vi "Reshape_DDcontroller.vi"(11 "path refs":path) -> (0 "error out":errorcluster, 3 "output array":dbl[](array[numeric]))   [LabVIEW 2021, in "System.lvclass"]
uses:
  System.lvclass
panel:
  out "Array":dbl[][](array[numeric])
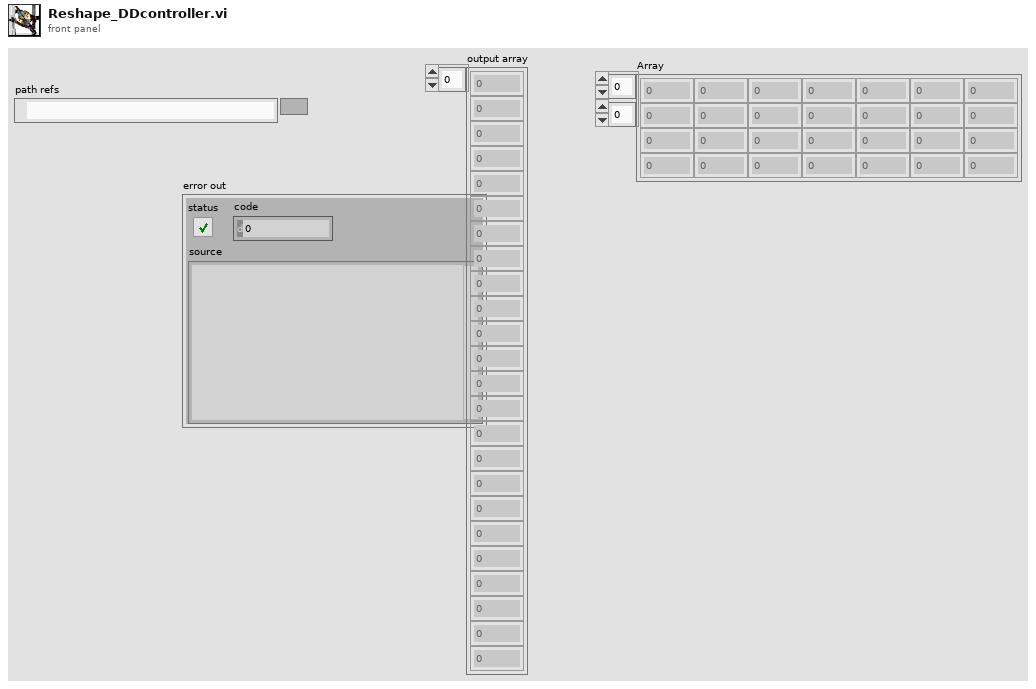
[diagram p1: front panel]
types:
  T1 = enum16{"big-endian, network order", "native, host order", "little-endian"}
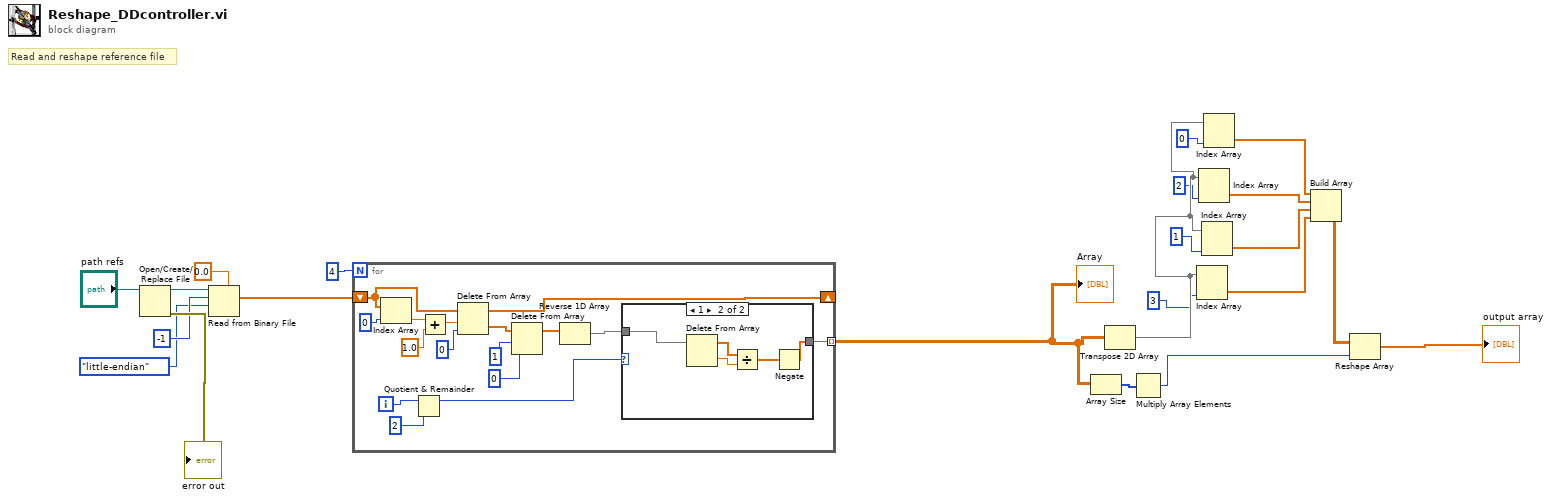
[diagram p0: block diagram]
diagram:
  # "Read and reshape reference file"
  n1 = Open/Create/Replace File(file path (use dialog)="path refs") -> (refnum out=w15:refnum<file>, error out=→"error out":errorcluster)  [unwired: 5 in, 1 out]
  n2 = Read from Binary File(5:0.0, 9:T1."little-endian" ("byte order (0:big-endian, network order)"), 10:-1 ("count (1)"), 11:w15) -> (2:w21:dbl[])  [unwired: 2 in, 3 out]
  n3 = for {
    N: 4 -> [_]
    shift-right: [w29] -> _
    shift-left: w21 -> [w35]
    tunnel: [w28] -> w7 mode=indexing
    i -> [w32]
    n4 = Index Array(array=w35, index=0 ("length")) -> (element=w36:dbl)
    n5 = Quotient & Remainder(x=w32, y=2) -> (x-y*floor(x/y)=w30:i32)  [unwired: 1 out]
    n6 = Add(x=w36, y=1.0) -> (x+y=w34:dbl)
    n7 = Delete From Array(array=w35, length=w34, index=0) -> (deleted portion=w24:dbl[], array with subset deleted=w29:dbl[])
    n8 = Delete From Array(array=w24, length=1, index=0) -> (array with subset deleted=w25:dbl[])  [unwired: 1 out]
    n9 = Reverse 1D Array(array=w25) -> (reversed array=w23:dbl[])
    n10 = case shown="1" w30 {
      tunnel: [w39 w41] -> w28
      tunnel: w23 -> [w39 w40]
      frame 0, Default {
      }
      frame 1 {
        n11 = Delete From Array(array=w40) -> (deleted portion=w43:dbl, array with subset deleted=w44:dbl[])  [unwired: 2 in]
        n12 = Divide(x=w44, y=w43) -> (x/y=w42:dbl[])
        n13 = Negate(x=w42) -> (-x=w41:dbl[])
      }
    }
  }
  "Array" <- w7
  n14 = Array Size(array=w7) -> (size(s)=w14:i32[])
  n15 = Transpose 2D Array(2D array=w7) -> (transposed array=w6:dbl[][])
  n16 = Multiply Array Elements(1:w14) -> (0:w8:i32)
  n17 = Index Array(array=w6, index (col)=3 ("index (row)")) -> (element=w9:dbl[])  [unwired: 1 in]
  n18 = Index Array(array=w6, index (col)=2 ("index (row)")) -> (element=w11:dbl[])  [unwired: 1 in]
  n19 = Index Array(array=w6, index (col)=1 ("index (row)")) -> (element=w10:dbl[])  [unwired: 1 in]
  n20 = Index Array(array=w6, index (col)=0 ("index (row)")) -> (element=w12:dbl[])  [unwired: 1 in]
  n21 = Build Array(w12, w11, w10, w9) -> (w5:dbl[][])
  n22 = Reshape Array(w5, w8) -> (→"output array":dbl[])
